vi "Get_Latest_Build_From_Artifactory.vi"(7 "Repository":string="CIBuild_Centauro") -> (4 "Output Path":path, 6 "UI File Path":path, 8 "Build":string, 10 "MC File Path":path, 15 "Error Out 2":errorcluster)   [LabVIEW 2016, in "Centauro.lvlib"]
uses:
  Projects/Centauro.lvlib
  <vilib>/regexp/Match Regular Expression.xnode
  <vilib>/httpClient/LabVIEWHTTPClient.lvlib
  <vilib>/zip/NI_Unzip.lvlib
panel:
  in  "Error In":errorcluster
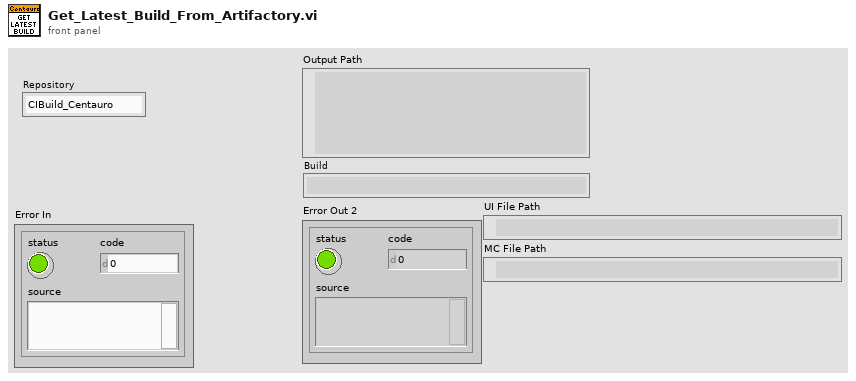
[diagram p1: front panel]
types:
  T1 = typedef "LabVIEWHTTPClient.lvlib/ClientHandle.ctl" = refnum<k1>
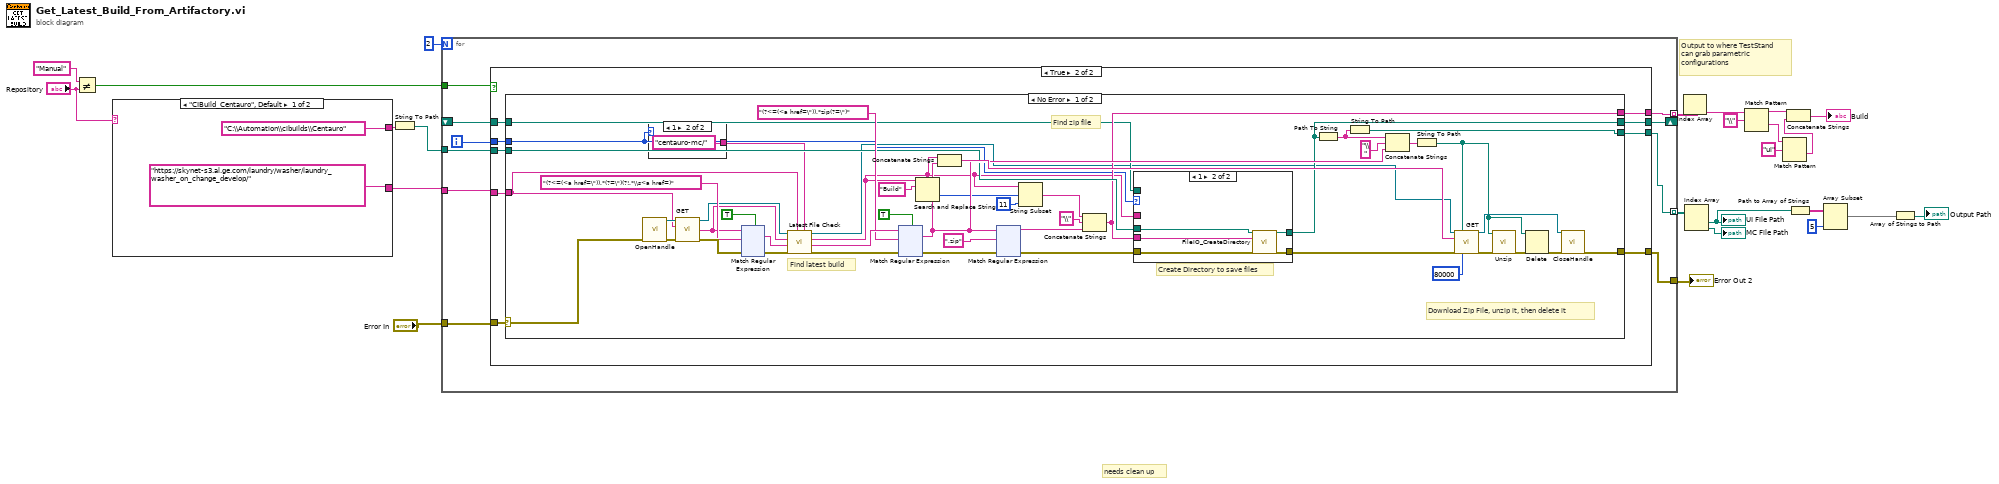
[diagram p0: block diagram]
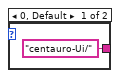
[diagram p3: hidden frame]
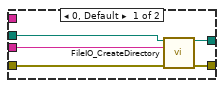
[diagram p4: hidden frame]
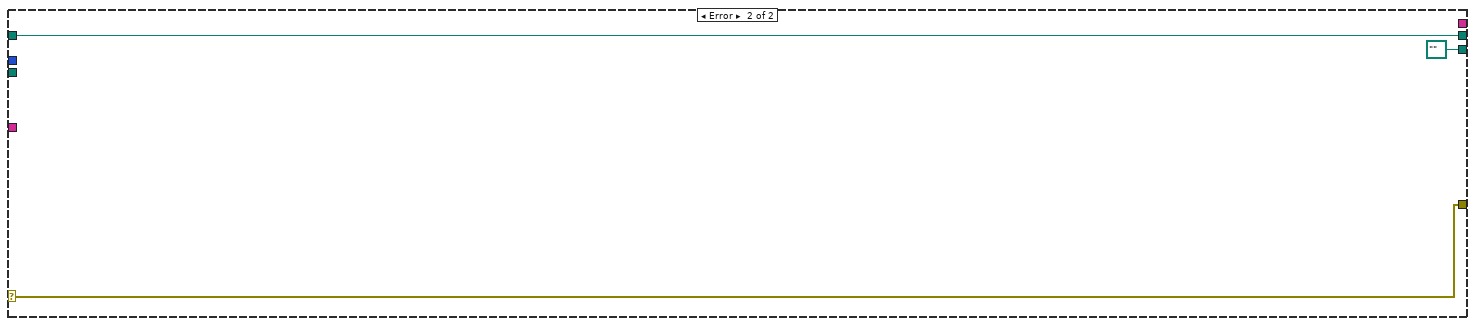
[diagram p5: hidden frame]
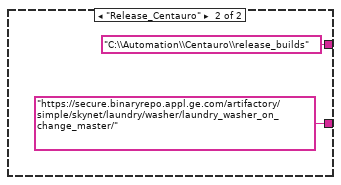
[diagram p6: hidden frame]
diagram:
  # "needs clean up"
  # "Output to where TestStand\ncan grab parametric\nconfigurations"
  n1 = Not Equal?(x="Manual" ("y"), y="Repository") -> (x != y?=w19:bool)
  n2 = case shown="\"CIBuild_Centauro\", Default" "Repository" {
    tunnel: ["C:\\Automation\\cibuilds\\Centauro" "C:\\Automation\\Centauro\\release_builds"] -> w15
    tunnel: ["https://skynet-s3.al.ge.com/laundry/washer/laundry_washer_on_change_develop/" ("regular expression") "https://secure.binaryrepo.appl.ge.com/artifactory/simple/skynet/laundry/washer/laundry_washer_on_change_master/" ("regular expression")] -> w16
    frame "CIBuild_Centauro", Default {
    }
    frame "Release_Centauro" {
    }
  }
  n3 = String To Path(string=w15) -> (path=w17:path)
  n4 = for {
    N: 2 -> [_]
    tunnel: w17 -> [w38]
    tunnel: w16 -> [w37]
    tunnel: [w36] -> w22 mode=indexing
    tunnel: [w35] -> w21
    tunnel: "Error In" -> [w34]
    shift-right: [w32] -> _
    shift-left: _ -> [w31]
    tunnel: w19 -> [w30]
    tunnel: [w29] -> w3 mode=indexing
    i -> [w33]
    n5 = case shown="True" w30 {
      tunnel: w37 -> [_ w49]
      tunnel: [_ w48] -> w29
      tunnel: [w40 w47] -> w35
      tunnel: w38 -> [_ w46]
      tunnel: [_ w45] -> w36
      tunnel: w34 -> [w40 w44]
      tunnel: w33 -> [_ w43]
      tunnel: [w39 w42] -> w32
      tunnel: w31 -> [w39 w41]
      frame False {
      }
      frame True {
        n6 = case shown="No Error" w44 {
          selector: w44 -> [w65 w452]
          tunnel: [w69 w452] -> w47
          tunnel: [w76 path ""] -> w48
          tunnel: w49 -> [w56 _]
          tunnel: w46 -> [w77 _]
          tunnel: [w66 _] -> w45
          tunnel: w43 -> [w54 _]
          tunnel: [w62 w450] -> w42
          tunnel: w41 -> [w61 w450]
          frame No Error {
            # "Find latest build"
            # "Create Directory to save files"
            # "Find zip file"
            # "Download Zip File, unzip it, then delete it"
            n7 = call <vilib>:"OpenHandle.vi"("error in (no error)"=w65) -> ("client handle out"=w94:T1, "error out"=w95:errorcluster)  [unwired: 13 in]
            n8 = case shown="1" w54 {
              tunnel: ["centauro-Ui/" ("string") "centauro-mc/" ("string")] -> w53
              frame 0, Default {
              }
              frame 1 {
              }
            }
            n9 = call <vilib>:"GET.vi"("client handle"=w94, "url"=w56, "error in (no error)"=w95) -> ("client handle out"=w60:T1, "body"=w58:string, "error out"=w93:errorcluster)  [unwired: 9 in, 1 out]
            n10 = xnode "Match Regular Expression"("input string"=w58, "regular expression"="(?<=(<a href=\")).*(?=\")(?!.*\\s<a href=)", "error in"=w93, "multiline? (F)"=TRUE) -> ("whole match"=w59:string, "error out"=w90:errorcluster)  [unwired: 2 in, 3 out]
            n11 = call "Latest File Check.vi"("Target File Path"=w53, "Initial File Path"=w56, "error in (no error)"=w90, "Matched Folder"=w59, "Initial body in"=w58, "Refnum in"=w60) -> ("error out"=w88:errorcluster, "body out"=w87:string, "File Path Out"=w57:string, "Refnum out"=w51:T1)  [unwired: 2 in]
            n12 = xnode "Match Regular Expression"("input string"=w87, "regular expression"="(?<=(<a href=\")).*zip(?=\")", "error in"=w88, "multiline? (F)"=TRUE) -> ("whole match"=w81:string, "error out"=w83:errorcluster)  [unwired: 2 in, 3 out]
            n13 = Search and Replace String(input string=w57, search string="Build") -> (offset past replacement=w72:i32)  [unwired: 6 in, 3 out]
            n14 = Concatenate Strings(w57, w81) -> (w85:string)
            n15 = xnode "Match Regular Expression"("input string"=w81, "regular expression"=".zip", "error in"=w83) -> ("before match"=w52:string, "error out"=w82:errorcluster)  [unwired: 3 in, 3 out]
            n16 = String Subset(string=w57, offset (0)=w72, length (rest)=11 ("length (rest)")) -> (substring=w71:string)
            n17 = Concatenate Strings(w71, "\\" ("string"), w52) -> (w66:string)
            n18 = case shown="1" w54 {
              tunnel: [w102 w103] -> w50
              tunnel: w82 -> [w101 w104]
              tunnel: w77 -> [w100 w107]
              tunnel: [w99 w105] -> w62
              tunnel: w66 -> [w98 w106]
              tunnel: w61 -> [_ _]
              tunnel: w57 -> [_ _]
              frame 0, Default {
                n19 = call "FileIO_CreateDirectory.vi"("Base Path"=w100, "Directory Name"=w98, "Error In"=w101) -> ("File Path Control"=w99:path, "Error Out"=w102:errorcluster)  [unwired: 11 in]
              }
              frame 1 {
                n20 = call "FileIO_CreateDirectory.vi"("Base Path"=w107, "Directory Name"=w106, "Error In"=w104) -> ("File Path Control"=w105:path, "Error Out"=w103:errorcluster)  [unwired: 11 in]
              }
            }
            n21 = Path To String(path=w62) -> (string=w64:string)
            n22 = String To Path(string=w64) -> (path=w76:path)
            n23 = Concatenate Strings(w64, "\\" ("string"), w81) -> (w79:string)
            n24 = String To Path(string=w79) -> (path=w63:path)
            n25 = call <vilib>:"GET.vi"("client handle"=w51, "output file"=w63, "url"=w85, "error in (no error)"=w50, "timeout (10000)"=80000) -> ("client handle out"=w67:T1, "error out"=w68:errorcluster)  [unwired: 7 in, 2 out]
            n26 = call <vilib>:"Unzip.vi"("error in (no error)"=w68, "Zip file"=w63) -> ("error out"=w78:errorcluster)  [unwired: 7 in, 2 out]
            n27 = Delete(path (use dialog)=w63, error in=w78) -> (error out=w55:errorcluster)  [unwired: 3 in, 2 out]
            n28 = call <vilib>:"CloseHandle.vi"("client handle"=w67, "error in (no error)"=w55) -> ("error out"=w69:errorcluster)  [unwired: 13 in]
          }
          frame Error {
          }
        }
      }
    }
  }
  "Error Out 2" <- w21
  n29 = Index Array(array=w22) -> (element=w14:string)  [unwired: 1 in]
  n30 = Index Array(array=w3) -> (element #1=w1:path, element #2=→"MC File Path":path)  [unwired: 2 in]
  "UI File Path" <- w1
  n31 = Match Pattern(string=w14, regular expression="\\") -> (before substring=w12:string, after substring=w11:string)  [unwired: 1 in, 2 out]
  n32 = Match Pattern(string=w11, regular expression="ui") -> (after substring=w9:string)  [unwired: 1 in, 3 out]
  n33 = Concatenate Strings(w12, w9) -> (→"Build":string)
  n34 = Path to Array of Strings(0:w1) -> (2:w7:string[])  [unwired: 1 out]
  n35 = Array Subset(array=w7, length=5) -> (w5:string[])  [unwired: 1 in]
  n36 = Array of Strings to Path(0:w5) -> (2:→"Output Path":path)  [unwired: 1 in]
